vi "DetectorOnly.vi"() -> ()   [LabVIEW 2014]
uses:
  <vilib>/FieldPoint/Polymorphic Write.llb/FP Write (Float -IO).vi
panel:
  out "IC Cathode Error":errorcluster caption="error out"
  out "IC Anode Error":errorcluster caption="error out"
  out "PGAC Cathode Error":errorcluster caption="error out"
  out "PGAC Anode Error":errorcluster caption="error out"
  in  "stop":bool
  in  "IC - readback V":dbl min=0.0 max=1000.0 step=1.0
  in  "IC CATHODE":dbl min=0.0 max=1000.0 step=1.0
  in  "IC + readback V":dbl min=0.0 max=1000.0 step=1.0
  in  "IC ANODE":dbl min=0.0 max=1000.0 step=1.0
  in  "PGAC - readback V":dbl min=0.0 max=1000.0 step=1.0
  in  "PGAC CATHODE":dbl min=0.0 max=1000.0 step=1.0
  in  "PGAC + readback V":dbl min=0.0 max=1000.0 step=1.0
  in  "PGAC ANODE":dbl min=0.0 max=1000.0 step=1.0
  # "If one or more voltages trips,\nmanually reset both values to Zero."
  # "Error messages ->"
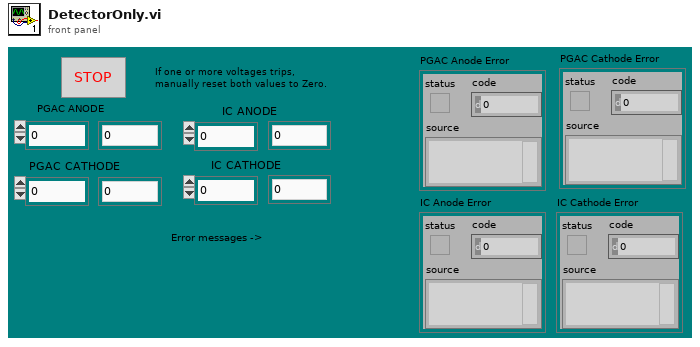
[diagram p1: front panel]
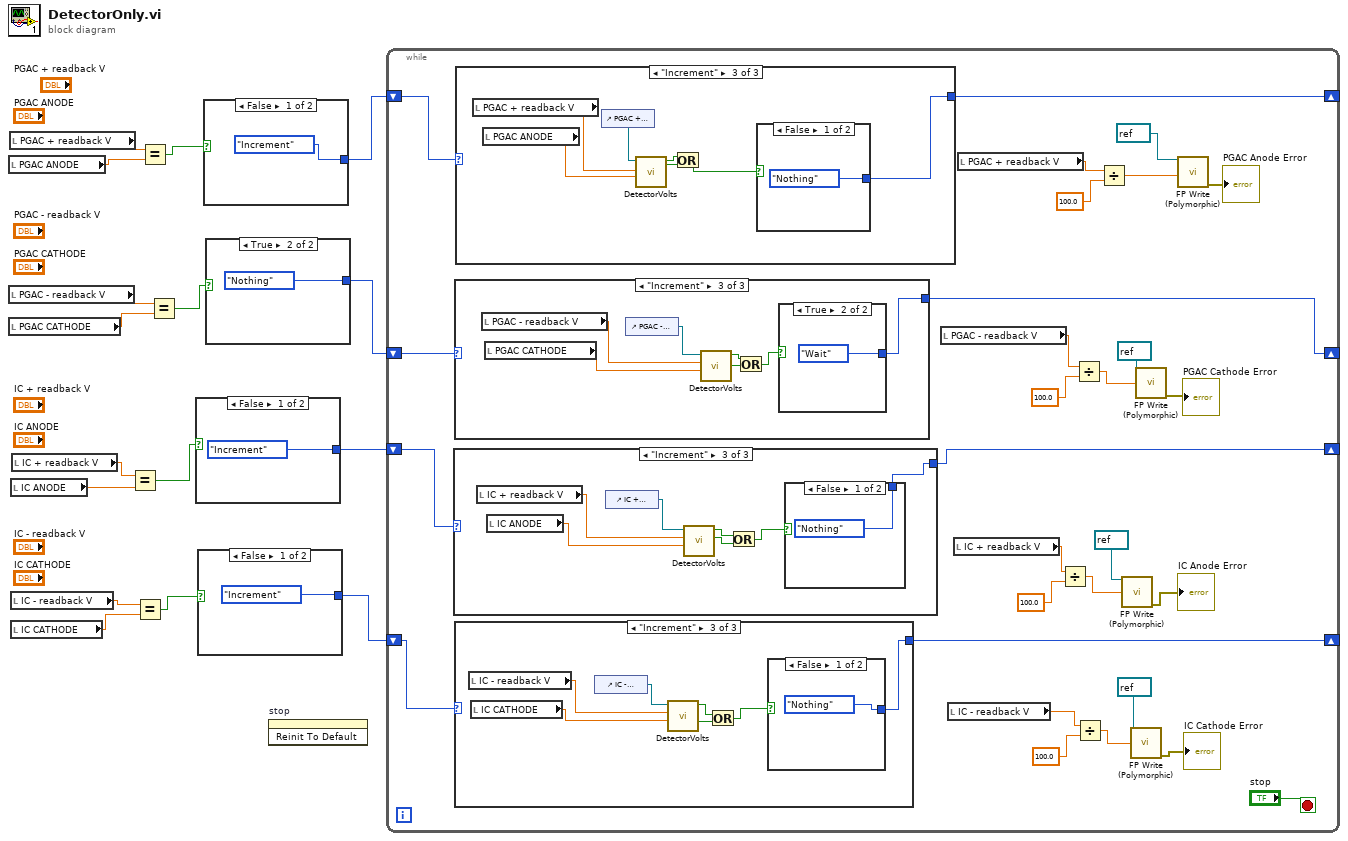
[diagram p0: block diagram]
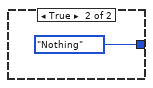
[diagram p2: hidden frame]
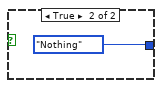
[diagram p3: hidden frame]
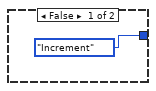
[diagram p4: hidden frame]
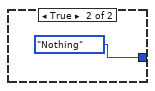
[diagram p5: hidden frame]
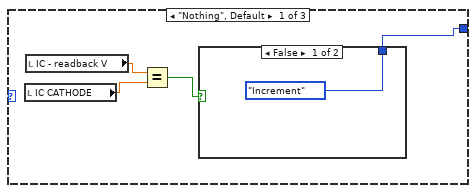
[diagram p6: hidden frame]
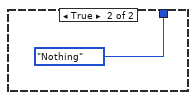
[diagram p7: hidden frame]
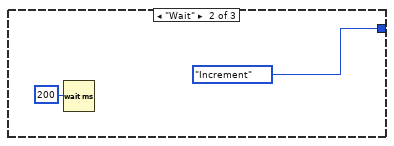
[diagram p8: hidden frame]
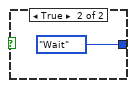
[diagram p9: hidden frame]
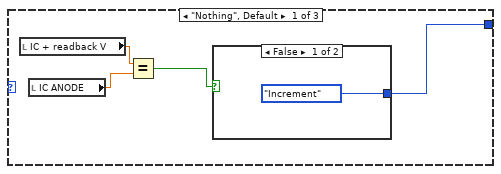
[diagram p10: hidden frame]
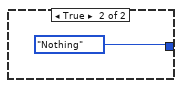
[diagram p11: hidden frame]
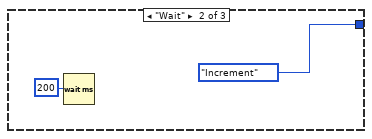
[diagram p12: hidden frame]
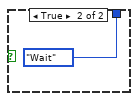
[diagram p13: hidden frame]
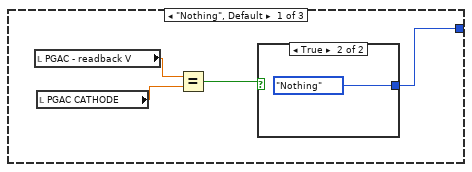
[diagram p14: hidden frame]
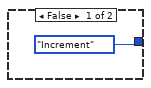
[diagram p15: hidden frame]
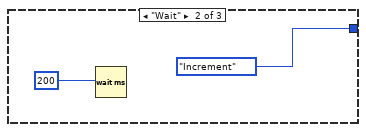
[diagram p16: hidden frame]
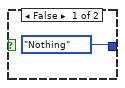
[diagram p17: hidden frame]
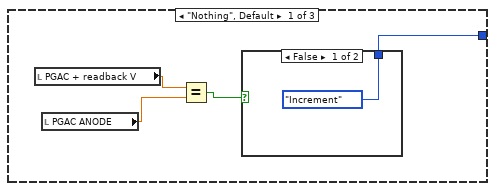
[diagram p18: hidden frame]
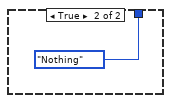
[diagram p19: hidden frame]
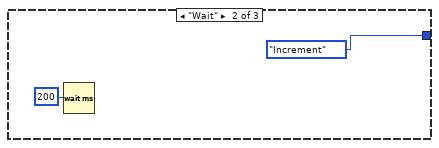
[diagram p20: hidden frame]
diagram:
  n1 = local read "PGAC ANODE"() -> (w10:dbl)
  n2 = local read "PGAC - readback V"() -> (w11:dbl)
  n3 = local read "PGAC CATHODE"() -> (w12:dbl)
  n4 = local read "PGAC + readback V"() -> (w9:dbl)
  n5 = local read "IC ANODE"() -> (w14:dbl)
  n6 = local read "IC - readback V"() -> (w15:dbl)
  n7 = local read "IC CATHODE"() -> (w16:dbl)
  n8 = local read "IC + readback V"() -> (w13:dbl)
  n9 = Equal?(x=w13, y=w14) -> (x = y?=w6:bool)
  n10 = Equal?(x=w15, y=w16) -> (x = y?=w5:bool)
  n11 = Equal?(x=w9, y=w10) -> (x = y?=w8:bool)
  n12 = Equal?(x=w11, y=w12) -> (x = y?=w7:bool)
  n13 = case shown="False" w6 {
    tunnel: [enum16{"Nothing", "Wait", "Increment"}."Increment" enum16{"Nothing", "Wait", "Increment"}."Nothing"] -> w2
    frame False {
    }
    frame True {
    }
  }
  n14 = case shown="False" w5 {
    tunnel: [enum16{"Nothing", "Wait", "Increment"}."Increment" enum16{"Nothing", "Wait", "Increment"}."Nothing"] -> w1
    frame False {
    }
    frame True {
    }
  }
  n15 = case shown="False" w8 {
    tunnel: [enum16{"Nothing", "Wait", "Increment"}."Increment" enum16{"Nothing", "Wait", "Increment"}."Nothing"] -> w4
    frame False {
    }
    frame True {
    }
  }
  n16 = case shown="True" w7 {
    tunnel: [enum16{"Nothing", "Wait", "Increment"}."Increment" enum16{"Nothing", "Wait", "Increment"}."Nothing"] -> w3
    frame False {
    }
    frame True {
    }
  }
  n17 = invoke on="stop" class="Bool" method="Reinit To Default"() -> ()  [unwired: 3 in, 3 out]
  n18 = while {
    shift-right: [w51] -> _
    shift-left: w4 -> [w52]
    shift-right: [w38] -> _
    shift-left: w3 -> [w45]
    shift-right: [w30] -> _
    shift-left: w2 -> [w34]
    shift-right: [w28] -> _
    shift-left: w1 -> [w29]
    stop <- "stop" stop-if-true
    n19 = case shown="\"Increment\"" w34 {
      tunnel: [w72 enum16{"Nothing", "Wait", "Increment"}."Increment" w81] -> w30
      frame "Nothing", Default {
        n20 = local read "IC + readback V"() -> (w74:dbl)
        n21 = local read "IC ANODE"() -> (w71:dbl)
        n22 = Equal?(x=w74, y=w71) -> (x = y?=w73:bool)
        n23 = case shown="False" w73 {
          tunnel: [enum16{"Nothing", "Wait", "Increment"}."Increment" enum16{"Nothing", "Wait", "Increment"}."Nothing"] -> w72
          frame False {
          }
          frame True {
          }
        }
      }
      frame "Wait" {
        n24 = Wait (ms)(milliseconds to wait=200) -> ()  [unwired: 1 out]
      }
      frame "Increment" {
        n25 = local read "IC + readback V"() -> (w79:dbl)
        n26 = local read "IC ANODE"() -> (w85:dbl)
        n27 = control-ref of="IC + readback V"() -> (w80:refnum<vi>)
        n28 = call "DetectorVolts.vi"("Detector"=w85, "Detector +/- readback V"=w79, "Digital in"=w80) -> ("Boolean 2"=w83:bool, "Boolean"=w84:bool)  [unwired: 7 in]
        n29 = Or(x=w84, y=w83) -> (x .or. y?=w82:bool)
        n30 = case shown="False" w82 {
          tunnel: [enum16{"Nothing", "Wait", "Increment"}."Nothing" enum16{"Nothing", "Wait", "Increment"}."Wait"] -> w81
          frame False {
          }
          frame True {
          }
        }
      }
    }
    n31 = case shown="\"Increment\"" w45 {
      tunnel: [w88 enum16{"Nothing", "Wait", "Increment"}."Increment" w97] -> w38
      frame "Nothing", Default {
        n32 = local read "PGAC - readback V"() -> (w91:dbl)
        n33 = local read "PGAC CATHODE"() -> (w90:dbl)
        n34 = Equal?(x=w91, y=w90) -> (x = y?=w89:bool)
        n35 = case shown="True" w89 {
          tunnel: [enum16{"Nothing", "Wait", "Increment"}."Increment" enum16{"Nothing", "Wait", "Increment"}."Nothing"] -> w88
          frame False {
          }
          frame True {
          }
        }
      }
      frame "Wait" {
        n36 = Wait (ms)(milliseconds to wait=200) -> ()  [unwired: 1 out]
      }
      frame "Increment" {
        n37 = local read "PGAC - readback V"() -> (w101:dbl)
        n38 = local read "PGAC CATHODE"() -> (w102:dbl)
        n39 = control-ref of="PGAC - readback V"() -> (w96:refnum<vi>)
        n40 = call "DetectorVolts.vi"("Detector"=w102, "Detector +/- readback V"=w101, "Digital in"=w96) -> ("Boolean 2"=w99:bool, "Boolean"=w100:bool)  [unwired: 7 in]
        n41 = Or(x=w100, y=w99) -> (x .or. y?=w98:bool)
        n42 = case shown="True" w98 {
          tunnel: [enum16{"Nothing", "Wait", "Increment"}."Nothing" enum16{"Nothing", "Wait", "Increment"}."Wait"] -> w97
          frame False {
          }
          frame True {
          }
        }
      }
    }
    n43 = case shown="\"Increment\"" w29 {
      tunnel: [w54 enum16{"Nothing", "Wait", "Increment"}."Increment" w64] -> w28
      frame "Nothing", Default {
        n44 = local read "IC CATHODE"() -> (w56:dbl)
        n45 = local read "IC - readback V"() -> (w57:dbl)
        n46 = Equal?(x=w57, y=w56) -> (x = y?=w55:bool)
        n47 = case shown="False" w55 {
          tunnel: [enum16{"Nothing", "Wait", "Increment"}."Increment" enum16{"Nothing", "Wait", "Increment"}."Nothing"] -> w54
          frame False {
          }
          frame True {
          }
        }
      }
      frame "Wait" {
        n48 = Wait (ms)(milliseconds to wait=200) -> ()  [unwired: 1 out]
      }
      frame "Increment" {
        n49 = local read "IC - readback V"() -> (w68:dbl)
        n50 = local read "IC CATHODE"() -> (w67:dbl)
        n51 = control-ref of="IC - readback V"() -> (w63:refnum<vi>)
        n52 = call "DetectorVolts.vi"("Detector"=w67, "Detector +/- readback V"=w68, "Digital in"=w63) -> ("Boolean 2"=w62:bool, "Boolean"=w66:bool)  [unwired: 7 in]
        n53 = Or(x=w66, y=w62) -> (x .or. y?=w65:bool)
        n54 = case shown="False" w65 {
          tunnel: [enum16{"Nothing", "Wait", "Increment"}."Nothing" enum16{"Nothing", "Wait", "Increment"}."Wait"] -> w64
          frame False {
          }
          frame True {
          }
        }
      }
    }
    n55 = case shown="\"Increment\"" w52 {
      tunnel: [w105 enum16{"Nothing", "Wait", "Increment"}."Increment" w114] -> w51
      frame "Nothing", Default {
        n56 = local read "PGAC + readback V"() -> (w108:dbl)
        n57 = local read "PGAC ANODE"() -> (w107:dbl)
        n58 = Equal?(x=w108, y=w107) -> (x = y?=w106:bool)
        n59 = case shown="False" w106 {
          tunnel: [enum16{"Nothing", "Wait", "Increment"}."Increment" enum16{"Nothing", "Wait", "Increment"}."Nothing"] -> w105
          frame False {
          }
          frame True {
          }
        }
      }
      frame "Wait" {
        n60 = Wait (ms)(milliseconds to wait=200) -> ()  [unwired: 1 out]
      }
      frame "Increment" {
        n61 = local read "PGAC + readback V"() -> (w118:dbl)
        n62 = local read "PGAC ANODE"() -> (w119:dbl)
        n63 = control-ref of="PGAC + readback V"() -> (w113:refnum<vi>)
        n64 = call "DetectorVolts.vi"("Detector"=w119, "Detector +/- readback V"=w118, "Digital in"=w113) -> ("Boolean 2"=w117:bool, "Boolean"=w116:bool)  [unwired: 7 in]
        n65 = Or(x=w116, y=w117) -> (x .or. y?=w115:bool)
        n66 = case shown="False" w115 {
          tunnel: [enum16{"Nothing", "Wait", "Increment"}."Nothing" enum16{"Nothing", "Wait", "Increment"}."Wait"] -> w114
          frame False {
          }
          frame True {
          }
        }
      }
    }
    n67 = local read "PGAC - readback V"() -> (w36:dbl)
    n68 = local read "IC - readback V"() -> (w25:dbl)
    n69 = local read "IC + readback V"() -> (w32:dbl)
    n70 = local read "PGAC + readback V"() -> (w49:dbl)
    n71 = Divide(x=w32, y=100.0) -> (x/y=w31:dbl)
    n72 = Divide(x=w36, y=100.0) -> (x/y=w35:dbl)
    n73 = Divide(x=w25, y=100.0) -> (x/y=w27:dbl)
    n74 = Divide(x=w49, y=100.0) -> (x/y=w48:dbl)
    n75 = call-poly <vilib>:"FP Write (Polymorphic).vi"("FieldPoint IO Point In"=refnum<k21> refnum, "value"=w31) -> ("error out"=→"IC Anode Error":errorcluster)  [unwired: 11 in, 2 out]
    n76 = call-poly <vilib>:"FP Write (Polymorphic).vi"("FieldPoint IO Point In"=refnum<k21> refnum, "value"=w27) -> ("error out"=→"IC Cathode Error":errorcluster)  [unwired: 11 in, 2 out]
    n77 = call-poly <vilib>:"FP Write (Polymorphic).vi"("FieldPoint IO Point In"=refnum<k21> refnum, "value"=w35) -> ("error out"=→"PGAC Cathode Error":errorcluster)  [unwired: 11 in, 2 out]
    n78 = call-poly <vilib>:"FP Write (Polymorphic).vi"("FieldPoint IO Point In"=refnum<k21> refnum, "value"=w48) -> ("error out"=→"PGAC Anode Error":errorcluster)  [unwired: 11 in, 2 out]
  }
